vi "Get Formatter.vi"(8 "error in (no error)":errorcluster, 11 "Endpoint in":refnum<class "Endpoint.lvclass">) -> (0 "error out":errorcluster, 2 "Format":refnum<class "Stream Formatter.lvclass">, 3 "Endpoint out":refnum<class "Endpoint.lvclass">)   [LabVIEW 2020, in "Stream-Simple-Msg.lvlib" / "Endpoint.lvclass"]
uses:
  Endpoint.lvclass
  Stream Formatter/Stream Formatter.lvclass
  Endpoint.lvclass/Endpoint.ctl
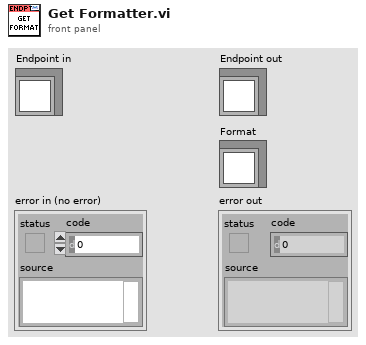
[diagram p1: front panel]
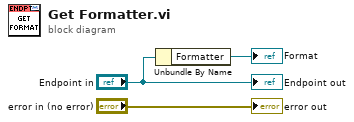
[diagram p0: block diagram]
diagram:
  n1 = Unbundle By Name("Endpoint in") -> ("Formatter"=→"Format":refnum<class "Stream Formatter.lvclass">)
  "error out" <- "error in (no error)"
  "Endpoint out" <- "Endpoint in"
